vi "Read Legend Minimum.vi"(9 "WaveformChart in":refnum<class "WaveformChart.lvclass">) -> (3 "WaveformChart out":refnum<class "WaveformChart.lvclass">, 4 "Legend Minimum":u32)   [LabVIEW 2014, in "WaveformChart.lvclass"]
uses:
  WaveformChart.lvclass
  WaveformChart.lvclass/WaveformChart.ctl
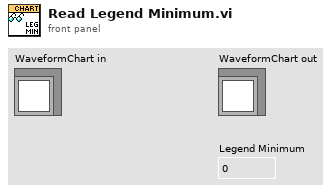
[diagram p1: front panel]
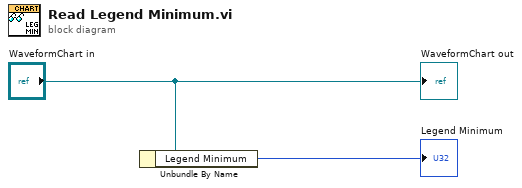
[diagram p0: block diagram]
diagram:
  n1 = Unbundle By Name("WaveformChart in") -> ("Legend Minimum"=→"Legend Minimum":u32)
  "WaveformChart out" <- "WaveformChart in"
